vi "Read Profiles(for High-Speed Data Communication).vi"(0 "Device ID (0)":i32, 5 "Timeout":u32, 11 "error in (no error)":errorcluster) -> (3 "Profile Info":T1, 4 "Device ID out":i32, 6 "Profile Data":u32[](array[numeric]), 8 "Rsp Profile Cnt":u32, 10 "Notify":u32, 14 "Buf Usage Rate":u32, 15 "error out":errorcluster)   [LabVIEW 2014, in "Keyence LJ-V7000.lvlib"]
doc: "Profile data will be acquired by high-speed communication.\nProfile data will be stored in a unit of 0.01 ƒÊm.\n\n<B>Note</B>:\nRefer to <B>10.3</B> in a manual of measuring instrument drivers for contents (storage order and size) of data to be stored in profile data."
uses:
  Keyence LJ-V7000.lvlib
  Clusters/Profile Info.ctl
  constant/Driver VI No.ctl
panel:
  # "(c) 2012 KEYENCE CORPORATION.  ALL RIGHTS RESERVED."
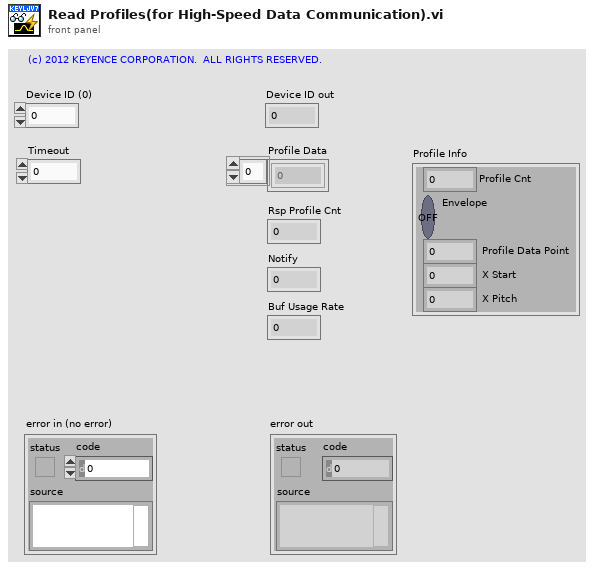
[diagram p1: front panel]
types:
  T1 = typedef "Keyence LJ-V7000.lvlib/Profile Info.ctl" = cluster{"Profile Cnt":u8, "Envelope":bool, " Profile Data Point":u16, " X Start":i32, " X Pitch":i32}
  T2 = typedef "Keyence LJ-V7000.lvlib/Driver VI No.ctl" = enum16{"Initialize", "Close", "Reboot Controller", "Return to Factory State", "Get System Error", "Clear System Error", "Trigger", "Start Batch Measurements", "Stop Batch Measurements", "Auto Zero", "Timing", "Reset", "Clear Memory", "Set Setting", "Get Setting", "Initialize Setting", "Reflect Setting", "Update Write Settings Area", "Check Status of Saving to Save Area", "Set Time", "Get Time", "Change Program", "Read Active Program Number", "Read Measurement Data", "Read Profiles(for High-Speed Mode)", "Read Batch Profiles(for High-Speed Mode)", "Read Profiles(for Advanced Mode)", "Read Batch Profiles(for Advanced Mode)", "Start Storage", "Stop Storage", "Read Storage Status", "Read Data Storage Data", "Read Profile Storage Data", "Read Batch Profile Storage Data", "Start High-Speed Data Communication", "Stop High-Speed Data Communication", "Read Profiles(for High-Speed Communication)"}
  T3 = cluster{"Profile Cnt":u8, u8, "reserve":u8, "reserve":u8, " Profile Data Point":u16, "reserve":u8, "reserve":u8, " X Start":i32, " XPitch":i32}
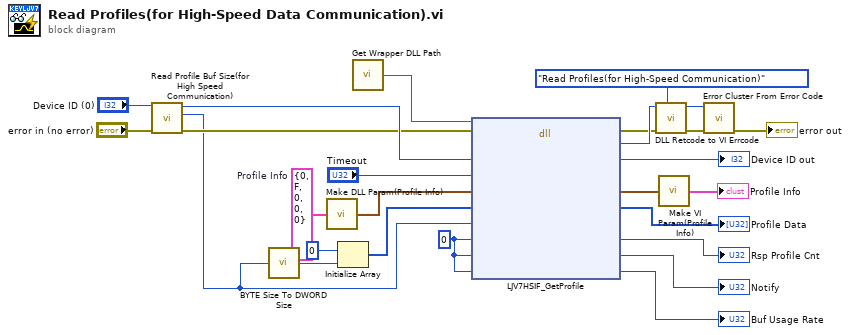
[diagram p0: block diagram]
diagram:
  w7 = u32 0 ("pdwRspProfileCnt")
  w23 = T1 {"Profile Cnt"=0, "Envelope"=FALSE, " Profile Data Point"=0, " X Start"=0, " X Pitch"=0}  # Profile Info
  n1 = call "Read Profile Buf Size(for High Speed Communication).vi"("error in (no error)"="error in (no error)", "Device ID (0)"="Device ID (0)") -> ("error out"=w15:errorcluster, "Profile Buf Size"=w8:u32, "Device ID out"=w17:i32)  [unwired: 7 in]
  n2 = call "BYTE Size To DWORD Size.vi"("BYTE Size"=w8) -> ("DWORD Size"=w9:u32)
  n3 = call "Make DLL Param(Profile Info).vi"("Profile Info"=w23) -> ("DLL Parameter"=w22:T3)
  n4 = Initialize Array(u32 0, w9) -> (w13:u32[])
  n5 = call "Get Wrapper DLL Path.vi"() -> ("Wrapper DLL Path"=w25:path)  [unwired: 1 in]
  n6 = dll-call lib="C:/Program Files/National Instruments/LabVIEW 2011/instr.lib/Keyence LJ-V7000/LJV7_HighSpeedWrapper.dll" fn="LJV7HSIF_GetProfile"(path in=w25, error in=w15, "lDeviceId"=w17, "dwTimeout"="Timeout", "pProfileInfo"=w22, "pdwData"=w13, "dwDataSize"=w8, "pdwRspProfileCnt"=w7, "pdwNotify"=w7, "pdwUsageRate"=w7) -> (error out=w3:errorcluster, "lRetCode"=w4:i32, "lDeviceId"=→"Device ID out":i32, "pProfileInfo"=w11:T3, "pdwData"=→"Profile Data":u32[], "pdwRspProfileCnt"=→"Rsp Profile Cnt":u32, "pdwNotify"=→"Notify":u32, "pdwUsageRate"=→"Buf Usage Rate":u32)  [unwired: 3 in, 1 out]
  n7 = call "DLL Retcode to VI Errcode.vi"("Driver VI No"=Driver_VI_No."Read Profiles(for High-Speed Communication)", "error in (no error)"=w3, "DLL Return Code"=w4) -> ("error out"=w6:errorcluster, "VI Error Code"=w5:i32)  [unwired: 7 in]
  n8 = call "Make VI Param(Profile Info).vi"("pProfileInfo"=w11) -> ("Profile Info"=→"Profile Info":T1)
  n9 = call <vilib>:"Error Cluster From Error Code.vi"("error in (no error)"=w6, "error code (0)"=w5) -> ("error out"=→"error out":errorcluster)  [unwired: 7 in]
